vi "Align and Subtract two Waveforms (continuous).vi"() -> ()   [LabVIEW 2020]
doc: "This example demonstrates the use of resampling and alignment to align two waveforms before subtracting one from the other. Aligning results in the waveforms being sampled at the same points in time."
uses:
  <vilib>/measure/maresamp.llb/Align two Waveforms (continuous).vi
  <vilib>/measure/NI_MABase.lvlib
  <vilib>/measure/NI_MAPro.lvlib
panel:
  in  "run state":bool=TRUE
  in  "frequency":dbl=3.0
  out "Aligned Waveforms and Difference Signal":waveform(dbl)[](graph)
  in  "delay waveform B":dbl(slide)=1.0082666666666666 scale=0.0..1.99
  in  "Stop":bool
  # "Overview: Demonstrates the use of resampling and alignment to align two waveforms before subtracting one from the other.\nRequirements: LabVIEW Full Development System\nInstructions:\n1. Run the VI. Observe that the signals are aligned to the same time stamp, then subtracted.\n2. Change the values of frequency and delay waveform B and observe the change in the graph.\n3. Click the run state button to reset the resampling and alignment calculations.\n4. Click Stop to stop the VI."
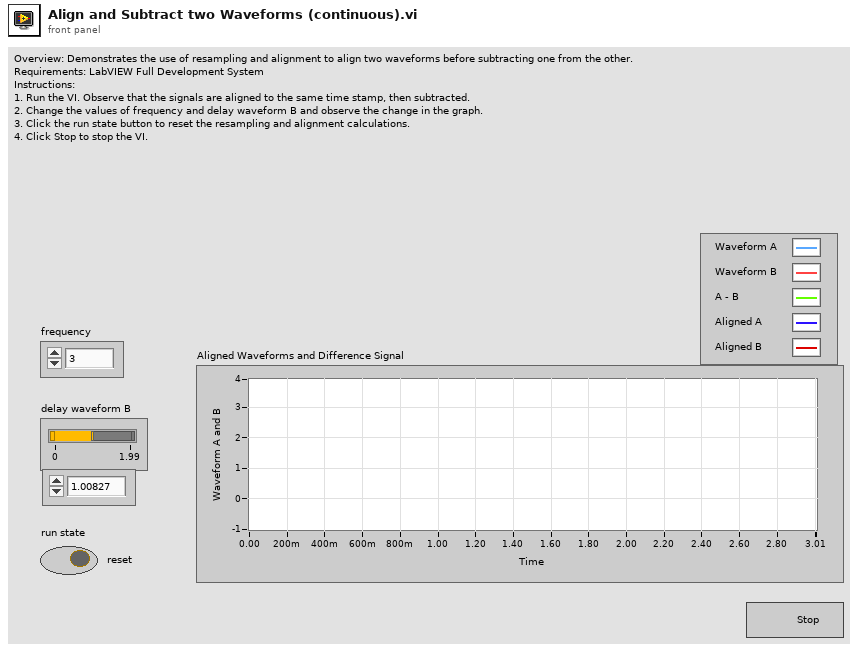
[diagram p1: front panel]
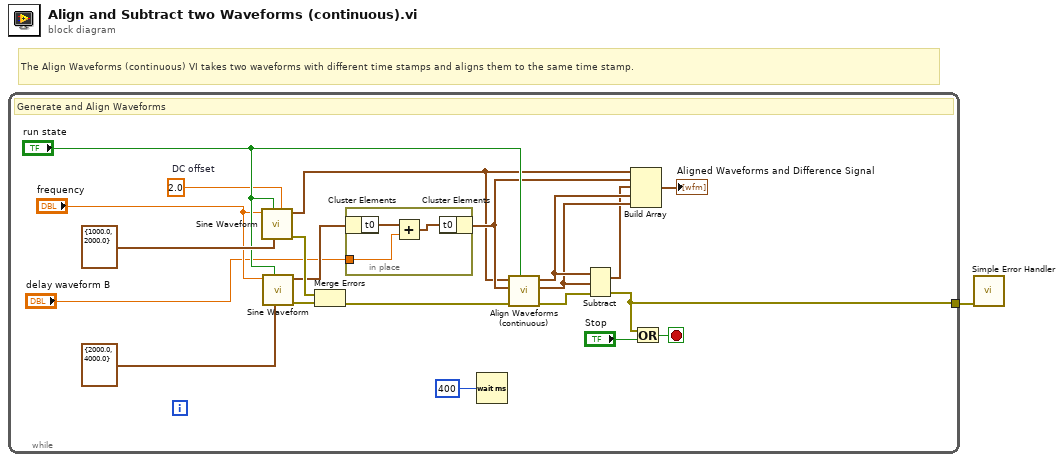
[diagram p0: block diagram]
diagram:
  # "The Align Waveforms (continuous) VI takes two waveforms with different time stamps and aligns them to the same time stamp."
  n1 = while {
    tunnel: [w9] -> w1
    stop <- w10 stop-if-true
    w4 = 2.0  # DC offset
    # "Generate and Align Waveforms"
    n2 = call <vilib>:"Sine Waveform.vi"("offset"=w4, "sampling info"=cluster{"Fs":dbl, "#s":dbl} {"Fs"=1000.0, "#s"=2000.0} ("sampling info A"), "reset signal"="run state", "frequency"="frequency") -> ("error out"=w12:errorcluster, "signal out"=w2:waveform(dbl))  [unwired: 3 in, 3 out]
    n3 = call <vilib>:"Sine Waveform.vi"("sampling info"=cluster{"Fs":dbl, "#s":dbl} {"Fs"=2000.0, "#s"=4000.0} ("sampling info B"), "reset signal"="run state", "frequency"="frequency") -> ("error out"=w13:errorcluster, "signal out"=w7:waveform(dbl))  [unwired: 4 in, 3 out]
    n4 = Merge Errors(w12, w13) -> (w11:errorcluster)
    n5 = in-place {
      in-place-border: "delay waveform B" -> [w23]
      n6 = in-place-cluster #1(w7) -> ("t0"=w25:timestamp)
      n7 = Add(x=w25, y=w23) -> (x+y=w24:timestamp)
      n8 = in-place-cluster #1("t0"=w24) -> (w6:waveform(dbl))
    }
    n9 = Wait (ms)(milliseconds to wait=u32 400) -> ()  [unwired: 1 out]
    n10 = call-poly <vilib>:"Align Waveforms (continuous).vi"("reset"="run state", "error in (no error)"=w11, "waveform B in"=w6, "waveform A in"=w2) -> ("error out"=w14:errorcluster, "waveform B out"=w15:waveform(dbl), "waveform A out"=w16:waveform(dbl))  [unwired: 3 in, 2 out]
    n11 = Subtract(1:w15, 2:w16, 4:w14) -> (0:w3:waveform(dbl), 3:w9:errorcluster)
    n12 = Build Array(w2, w6, w3, w16, w15) -> (→"Aligned Waveforms and Difference Signal":waveform(dbl)[])
    n13 = Or(x=w9, y="Stop") -> (x .or. y?=w10:bool)
  }
  n14 = call <vilib>:"Simple Error Handler.vi"("error in (no error)"=w1) -> ()  [unwired: 4 in, 5 out]
